vi "Write Alarm Message.vi"(8 "error in (no error)":errorcluster, 10 "alarm message":string, 11 "NT Base in":refnum<class "NT Base.lvclass">) -> (0 "error out":errorcluster, 3 "NT Base out":refnum<class "NT Base.lvclass">)   [LabVIEW 2020, in "PV Access.lvlib" / "PV Data.lvlib" / "NT Base.lvclass"]
uses:
  NT Base.lvclass
  NT Base.lvclass/NT Base.ctl
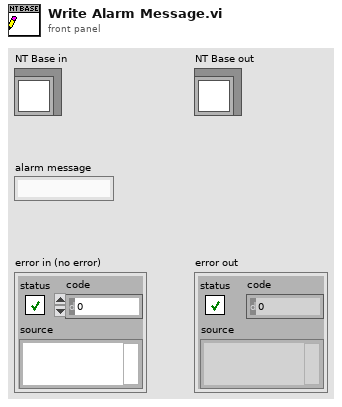
[diagram p1: front panel]
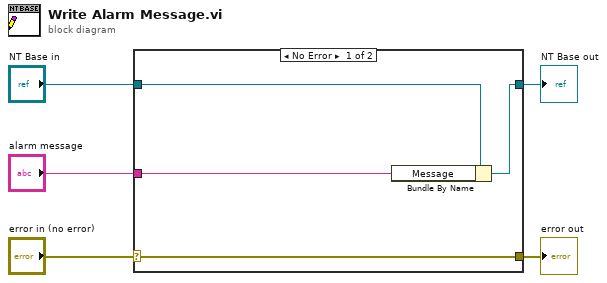
[diagram p0: block diagram]
diagram:
  n1 = case shown="No Error" "error in (no error)" {
    selector: "error in (no error)" -> [w9 w10]
    tunnel: [w9 w10] -> w4
    tunnel: [w7 w11] -> w2
    tunnel: "NT Base in" -> [w8 w11]
    tunnel: "alarm message" -> [w6 _]
    frame No Error {
      n2 = Bundle By Name(cluster=w8, "Message"=w6) -> (w7:refnum<class "NT Base.lvclass">)
    }
    frame Error {
    }
  }
  "error out" <- w4
  "NT Base out" <- w2
